vi "Get Item Location.vi"(6 "Authentication Header":T1[](array[typedef]), 8 "error in (no error)":errorcluster, 10 "Task GID":string) -> (0 "error out":errorcluster)   [LabVIEW 2016]
uses:
  <vilib>/addons/_JKI.lib/REST Client/classes/REST Client/HTTP Header.ctl
  <vilib>/addons/_JKI.lib/REST Client/classes/REST Client/REST Client.lvclass
panel:
  out "output array":cluster{string, "Response body":string}[](array[cluster])
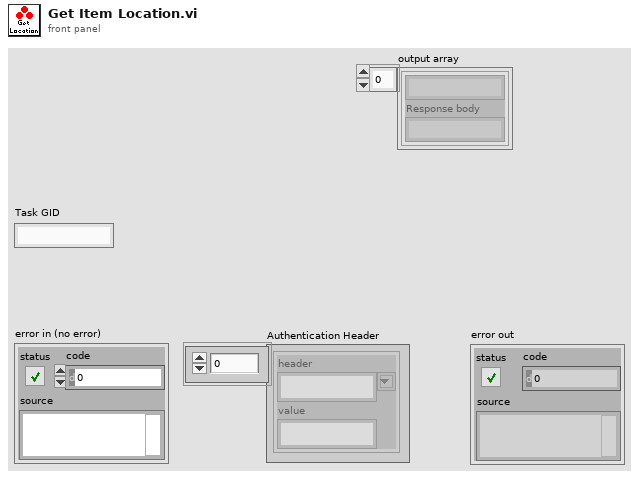
[diagram p1: front panel]
types:
  T1 = typedef "REST Client.lvlib/REST Client.lvclass/HTTP Header.ctl" = cluster{"header":string, "value":string}
  T2 = cluster{"Response body":string, "Response body":string}
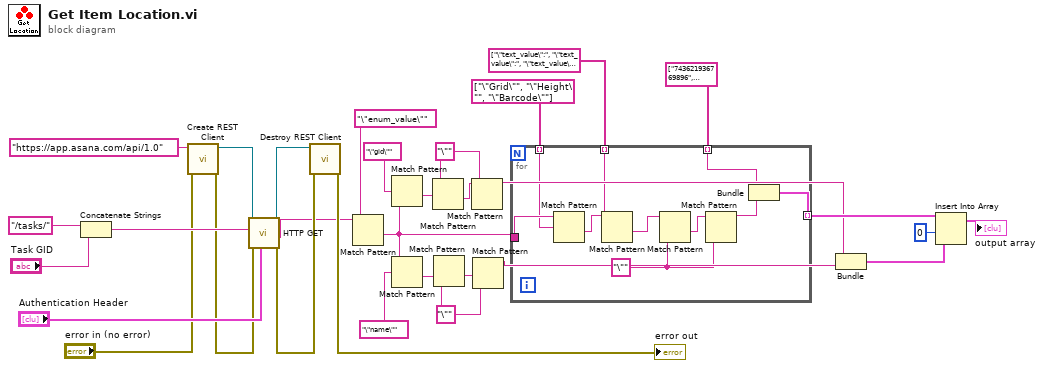
[diagram p0: block diagram]
diagram:
  w4 = "\""
  w3 = "\""
  n1 = Concatenate Strings("/tasks/", "Task GID") -> (w25:string)
  n2 = call <vilib>:"Create REST Client.vi"("error in (no error)"="error in (no error)", "Base URL"="https://app.asana.com/api/1.0") -> ("error out"=w23:errorcluster, "REST Client out"=w29:refnum<class "REST Client.lvclass">)  [unwired: 8 in]
  n3 = call-dynamic "HTTP GET.vi"("request specific headers"="Authentication Header", "error in (no error)"=w23, "Path"=w25, "REST Client in"=w29) -> ("error out"=w22:errorcluster, "Response body"=w18:string, "REST Client out"=w28:refnum<class "REST Client.lvclass">)  [unwired: 2 in, 3 out]
  n4 = call-dynamic "Destroy REST Client.vi"("error in (no error)"=w22, "REST Client in"=w28) -> ("error out"=→"error out":errorcluster)  [unwired: 9 in]
  n5 = Match Pattern(string=w18, regular expression="\"enum_value\"") -> (after substring=w12:string)  [unwired: 1 in, 3 out]
  n6 = Match Pattern(string=w12, regular expression="\"gid\"") -> (after substring=w1:string)  [unwired: 1 in, 3 out]
  n7 = Match Pattern(string=w12, regular expression="\"name\"") -> (after substring=w11:string)  [unwired: 1 in, 3 out]
  n8 = Match Pattern(string=w1, regular expression=w4) -> (after substring=w7:string)  [unwired: 1 in, 3 out]
  n9 = Match Pattern(string=w11, regular expression=w3) -> (after substring=w10:string)  [unwired: 1 in, 3 out]
  n10 = Match Pattern(string=w7, regular expression=w4) -> (before substring=w8:string)  [unwired: 1 in, 3 out]
  n11 = Match Pattern(string=w10, regular expression=w3) -> (before substring=w9:string)  [unwired: 1 in, 3 out]
  n12 = for {
    tunnel: string[] ["\"Grid\"", "\"Height\"", "\"Barcode\""] -> [w40] mode=indexing
    tunnel: w12 -> [w41]
    tunnel: string[] ["\"text_value\":", "\"text_value\":", "\"text_value\":"] -> [w38] mode=indexing
    tunnel: [w32] -> w15 mode=indexing
    tunnel: string[] ["743621936769896", "743912334990533", "505764283493351"] -> [w34] mode=indexing
    w36 = "\""
    n13 = Match Pattern(string=w41, regular expression=w40) -> (after substring=w39:string)  [unwired: 1 in, 3 out]
    n14 = Match Pattern(string=w39, regular expression=w38) -> (after substring=w37:string)  [unwired: 1 in, 3 out]
    n15 = Match Pattern(string=w37, regular expression=w36) -> (after substring=w35:string)  [unwired: 1 in, 3 out]
    n16 = Match Pattern(string=w35, regular expression=w36) -> (before substring=w33:string)  [unwired: 1 in, 3 out]
    n17 = Bundle(w34, "Response body"=w33) -> (w32:cluster{string, "Response body":string})  [unwired: 1 in]
  }
  n18 = Bundle("Response body"=w8, "Response body"=w9) -> (w6:T2)  [unwired: 1 in]
  n19 = Insert Into Array(array=w15, index=0, new element=w6) -> (→"output array":cluster{string, "Response body":string}[])
